vi "JTAG SPI.vi"(4 "Block Write Data":u8[](array[numeric]) format="%02x", 5 "Mask":u8=255 format="%02x", 6 "Blocksize":u16 format="%03x", 7 "Value":u8 format="%02x", 8 "error in (no error)":errorcluster, 9 "Target":u16(ring) items=["Power ASIC", "Stim ASIC", "MICS Radio", "FRAM"], 10 "Function":u16(ring) items=["Power UP", "Power DN", "Write Single", "Read Single", "Write Block", "Read Block", "Write Masked", "Test Value"], 11 "Address":u16 format="%04x") -> (0 "error out":errorcluster, 1 "Block Read Data":u16[](array[numeric]) format="%02x", 2 "Test Result":bool, 3 "Read Value":u8 format="%.0x")   [LabVIEW 2010]
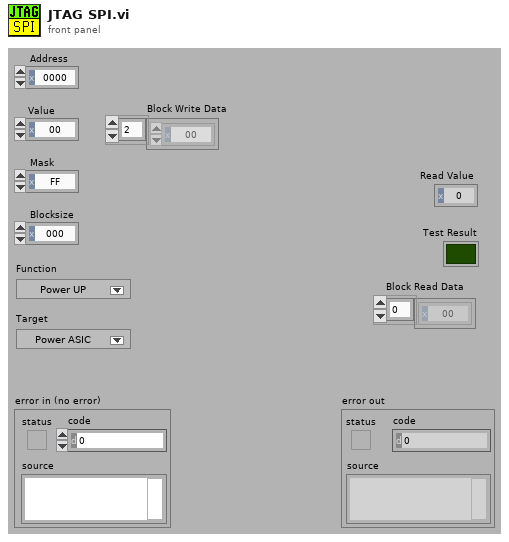
[diagram p1: front panel]
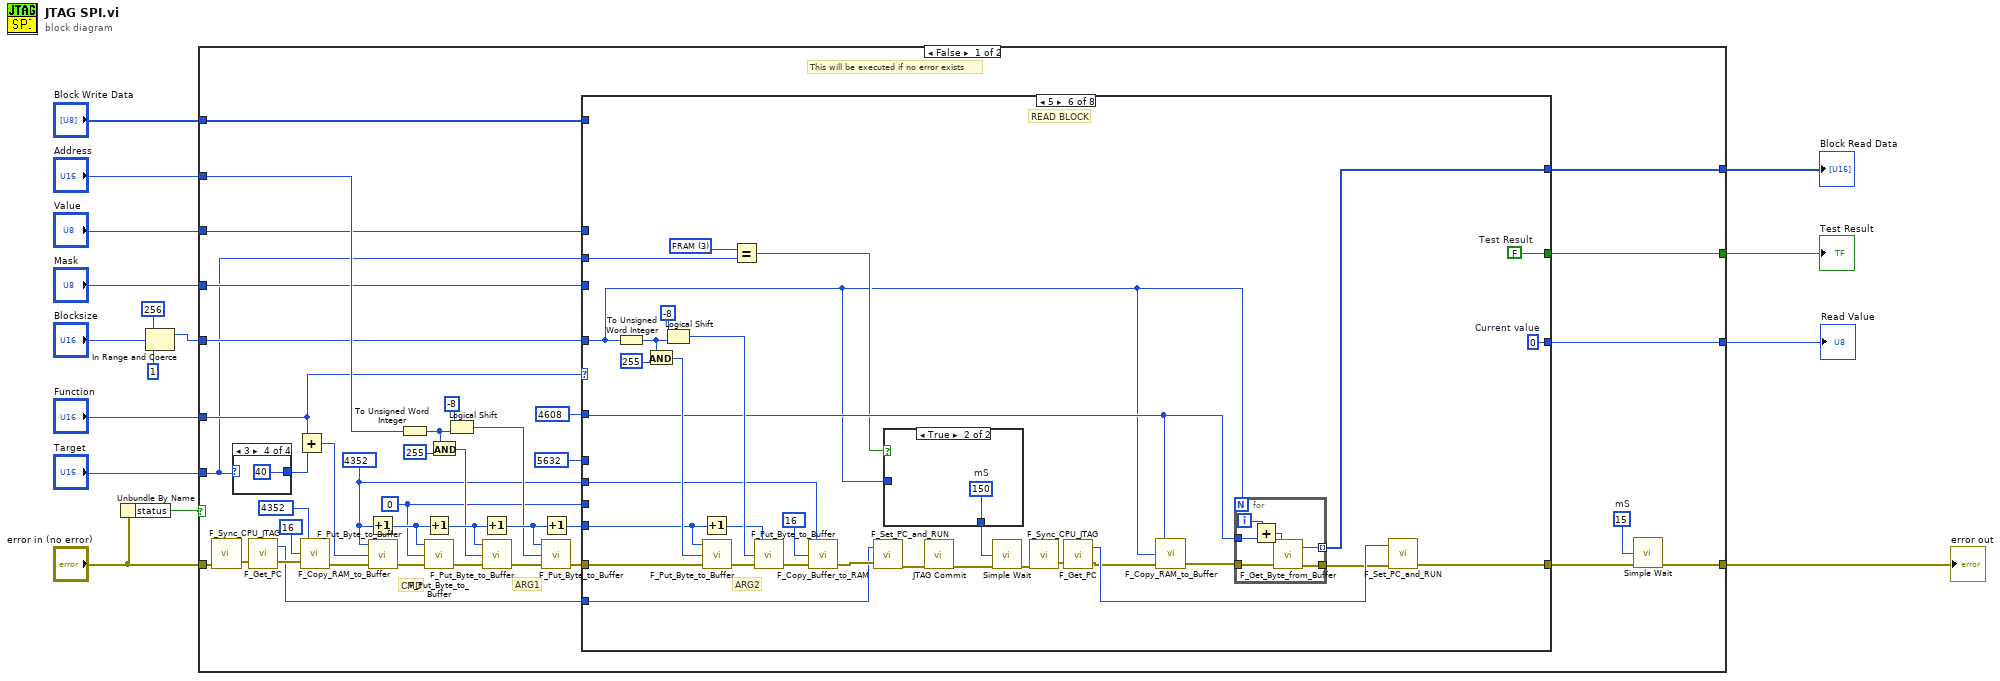
[diagram p0: block diagram]
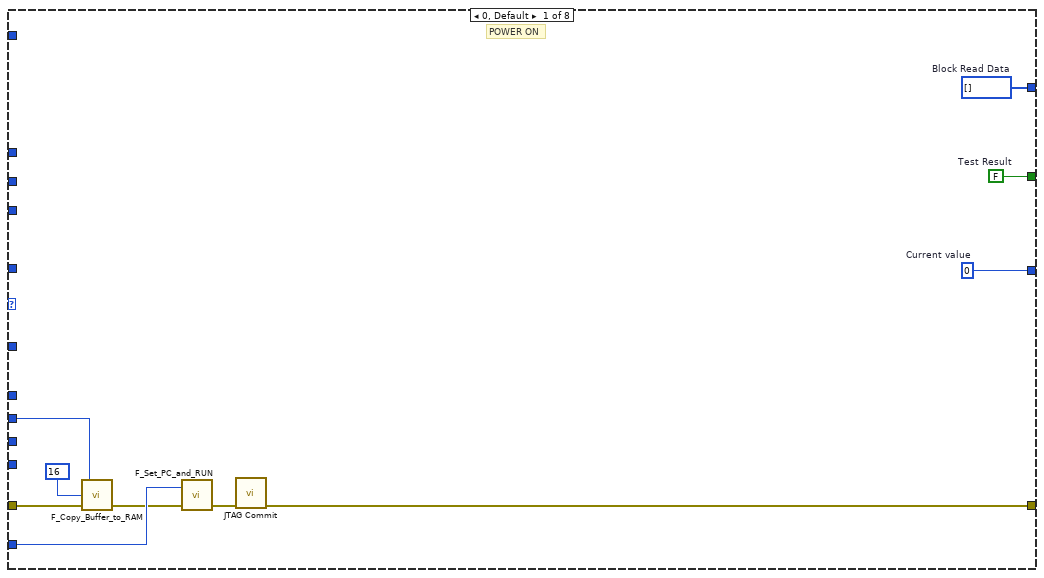
[diagram p2: hidden frame]
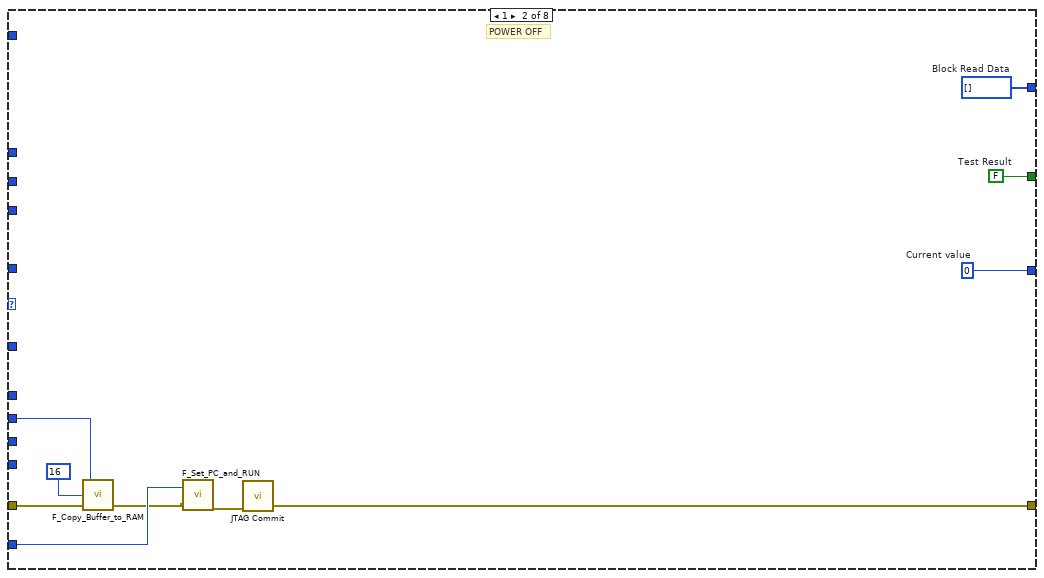
[diagram p3: hidden frame]
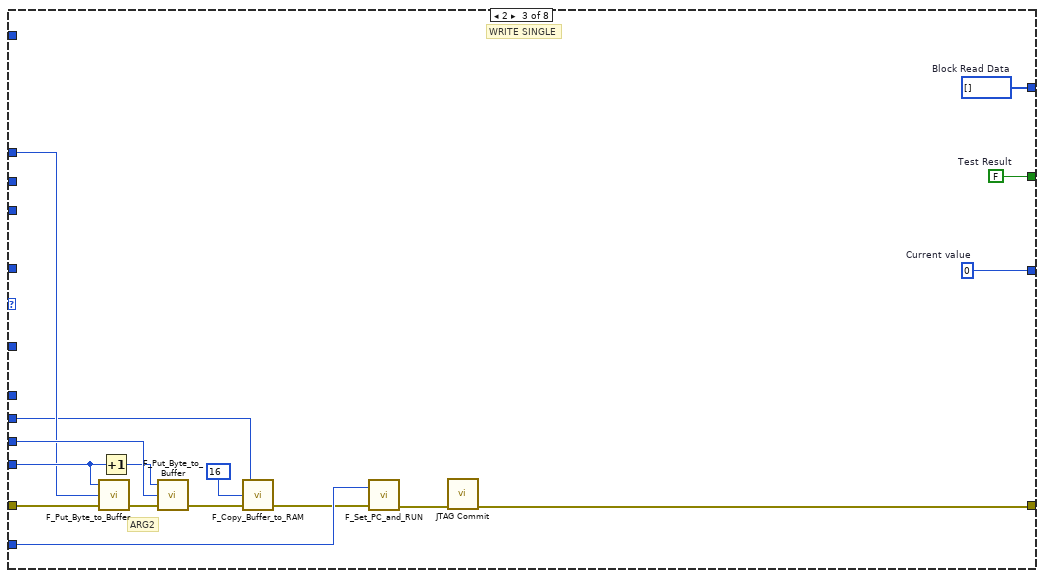
[diagram p4: hidden frame]
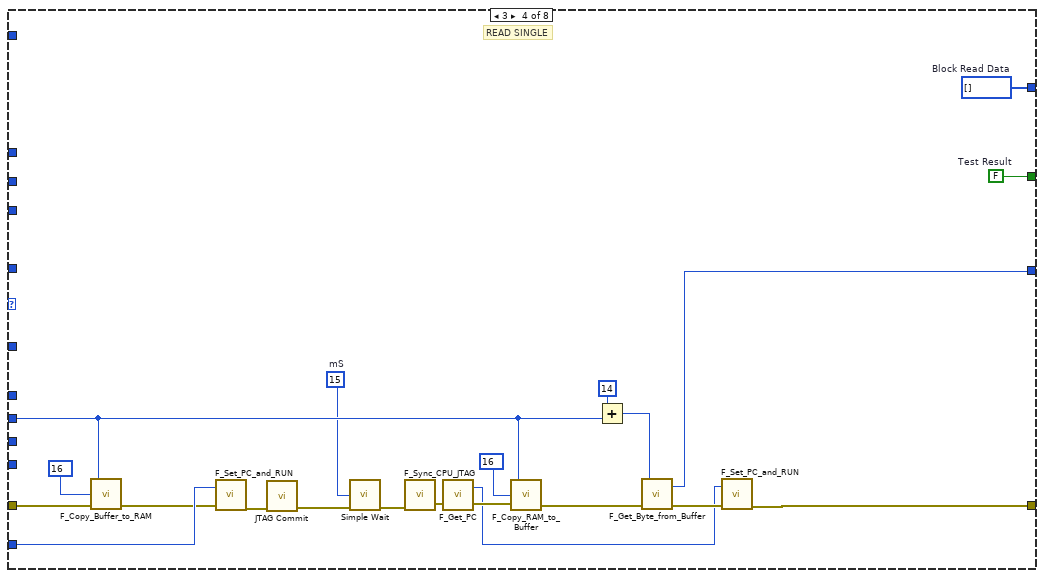
[diagram p5: hidden frame]
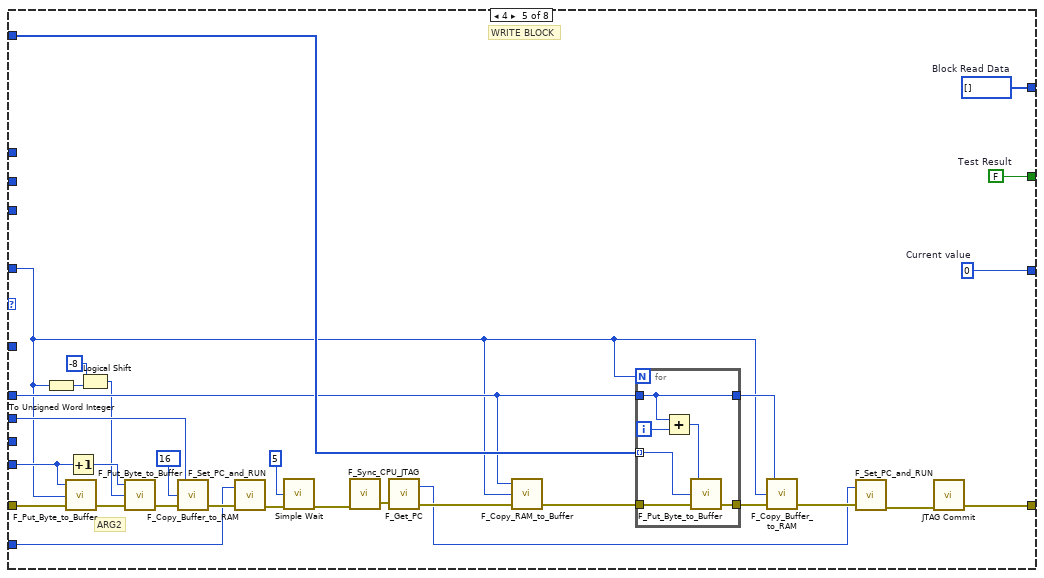
[diagram p6: hidden frame]
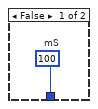
[diagram p7: hidden frame]
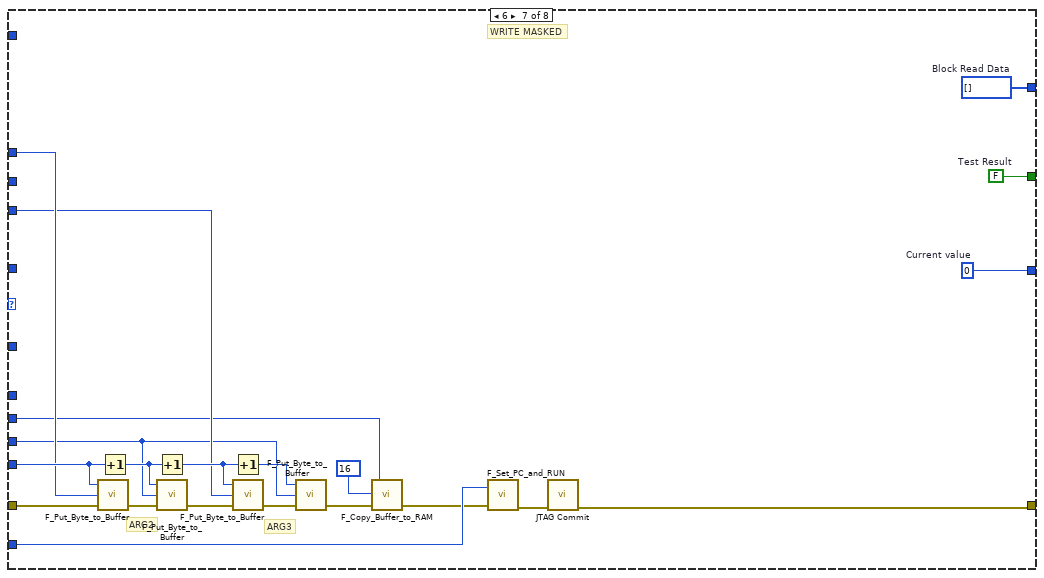
[diagram p8: hidden frame]
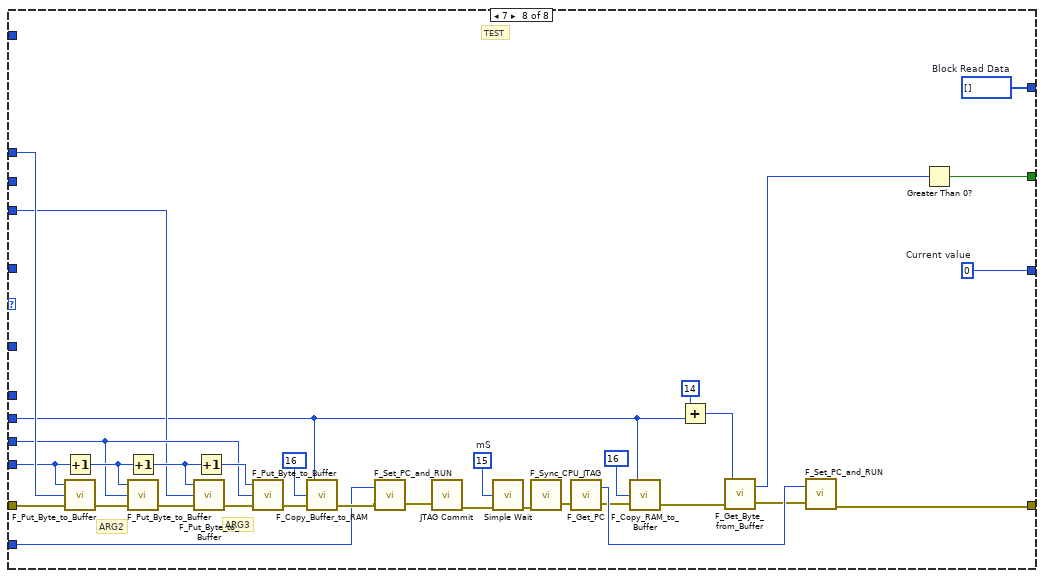
[diagram p9: hidden frame]
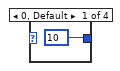
[diagram p10: hidden frame]
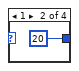
[diagram p11: hidden frame]
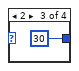
[diagram p12: hidden frame]
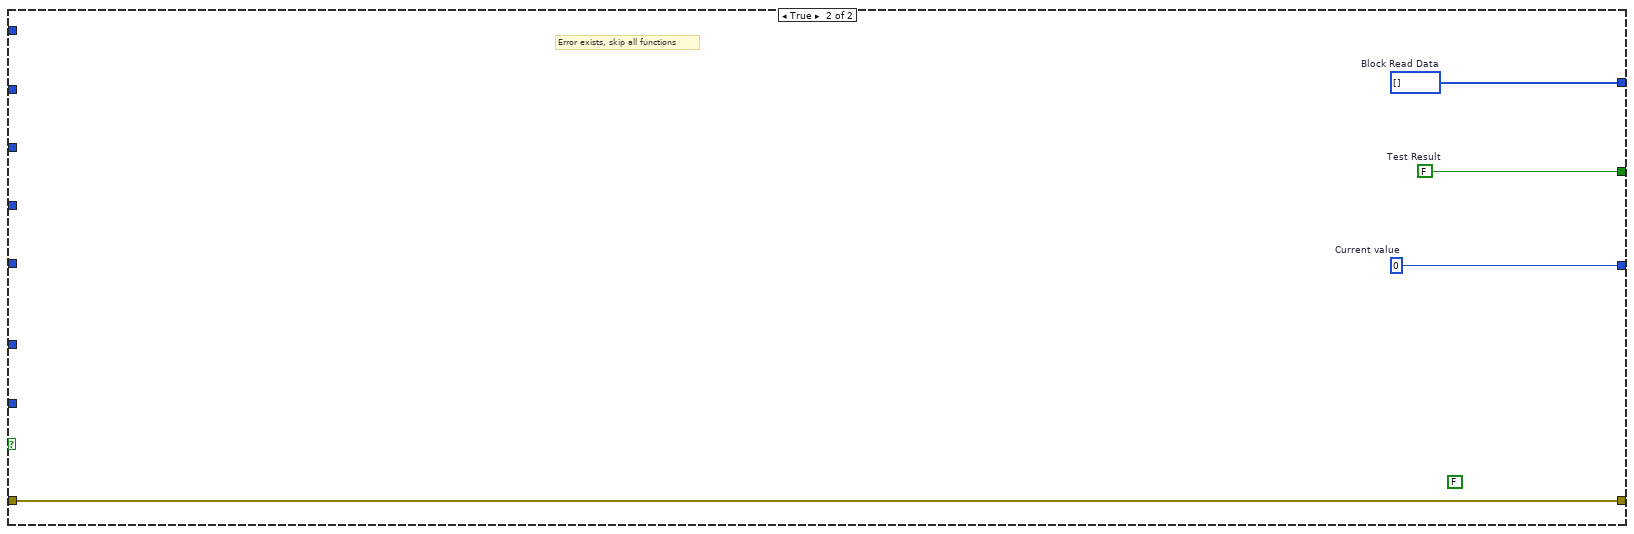
[diagram p13: hidden frame]
diagram:
  n1 = Unbundle By Name("error in (no error)") -> ("status"=w16:bool)
  n2 = In Range and Coerce(upper limit=u16 256, x="Blocksize", lower limit=u16 1) -> (coerced(x)=w4:u16)  [unwired: 1 out]
  n3 = case shown="False" w16 {
    tunnel: [w18 w250] -> w5
    tunnel: "error in (no error)" -> [w55 w250]
    tunnel: "Target" -> [w17 _]
    tunnel: "Address" -> [w44 _]
    tunnel: "Value" -> [w36 _]
    tunnel: "Mask" -> [w33 _]
    tunnel: w4 -> [w29 _]
    tunnel: "Function" -> [w21 _]
    tunnel: "Block Write Data" -> [w37 _]
    tunnel: [w35 w249] -> w7
    tunnel: [w34 w248] -> w8
    tunnel: [w30 w247] -> w6
    frame False {
      w20 = u32 15  # mS
      w38 = u16 0
      w32 = u16 4352
      # "ARG1"
      # "CMD"
      # "This will be executed if no error exists"
      n4 = call "F_Sync_CPU_JTAG.vi"("error in (no error)"=w55) -> ("error out"=w24:errorcluster)  [unwired: 1 in, 1 out]
      n5 = case shown="3" w17 {
        tunnel: [u16 10 u16 20 u16 30 u16 40] -> w54
        frame 0, Default {
        }
        frame 1 {
        }
        frame 2 {
        }
        frame 3 {
        }
      }
      n6 = call "F_Get_PC.vi"("error in (no error)"=w24) -> ("error out"=w23:errorcluster, "Program Counter"=w22:u16)  [unwired: 1 in]
      n7 = Add(x=w21, y=w54) -> (x+y=w53:u16)
      n8 = call "F_Copy_RAM_to_Buffer.vi"("error in (no error)"=w23, "Block size to be copied"=u16 16, "RAM start address"=u16 4352) -> ("error out"=w27:errorcluster)  [unwired: 2 in]
      n9 = Increment(x=w32) -> (x+1=w51:u16)
      n10 = call "F_Put_Byte_to_Buffer.vi"("error in (no error)"=w27, "New value"=w53, "Address of byte to be updated"=w32) -> ("error out"=w52:errorcluster)  [unwired: 2 in]
      n11 = To Unsigned Word Integer(number=w44) -> (unsigned 16bit integer=w41:u16)
      n12 = Increment(x=w51) -> (x+1=w48:u16)
      n13 = call "F_Put_Byte_to_Buffer.vi"("error in (no error)"=w52, "New value"=w38, "Address of byte to be updated"=w51) -> ("error out"=w50:errorcluster)  [unwired: 2 in]
      n14 = And(x=w41, y=u16 255) -> (x .and. y?=w45:u16)
      n15 = Logical Shift(y=i8 -8, x=w41) -> (x << y=w43:u16)
      n16 = Increment(x=w48) -> (x+1=w47:u16)
      n17 = call "F_Put_Byte_to_Buffer.vi"("error in (no error)"=w50, "New value"=w45, "Address of byte to be updated"=w48) -> ("error out"=w49:errorcluster)  [unwired: 2 in]
      n18 = Increment(x=w47) -> (x+1=w40:u16)
      n19 = call "F_Put_Byte_to_Buffer.vi"("error in (no error)"=w49, "New value"=w43, "Address of byte to be updated"=w47) -> ("error out"=w39:errorcluster)  [unwired: 2 in]
      n20 = case shown="5" w21 {
        tunnel: w40 -> [_ _ w87 _ w139 w174 w207 w231]
        tunnel: w39 -> [w60 w70 w89 w105 w141 w178 w208 w234]
        tunnel: w38 -> [_ _ w90 _ _ _ w197 w230]
        tunnel: w29 -> [_ _ _ _ w113 w149 _ _]
        tunnel: w37 -> [_ _ _ _ w134 _ _ _]
        tunnel: w36 -> [_ _ w86 _ _ _ w206 w232]
        tunnel: [w64 w74 w84 w111 w137 w170 w204 w240] -> w35
        tunnel: [w65 w75 w85 w112 w138 w180 w205 w223] -> w34
        tunnel: [w56 w66 w76 w92 w129 w153 w189 w210] -> w19
        tunnel: w33 -> [_ _ _ _ _ _ w198 w229]
        tunnel: w32 -> [w59 w68 w82 w108 w135 w164 w196 w224]
        tunnel: u16 5632 -> [_ _ _ _ w127 _ _ _]
        tunnel: w22 -> [w62 w72 w79 w110 w120 w162 w192 w221]
        tunnel: [w63 w73 w81 w106 w133 w171 w194 w238] -> w30
        tunnel: u16 4608 -> [_ _ _ _ _ w167 _ _]
        tunnel: w17 -> [_ _ _ _ _ w152 _ _]
        frame 0, Default {
          w63 = u8 0  # Current value
          w64 = u16[] []  # Block Read Data
          w65 = FALSE  # Test Result
          # "POWER ON"
          n21 = call "F_Copy_Buffer_to_RAM.vi"("error in (no error)"=w60, "Block size to be copied"=u16 16, "Buffer start address"=w59) -> ("error out"=w58:errorcluster)  [unwired: 2 in]
          n22 = call "F_Set_PC_and_RUN.vi"("error in (no error)"=w58, "PC start address"=w62) -> ("error out"=w57:errorcluster)  [unwired: 1 in]
          n23 = call "JTAG Commit.vi"("error in (no error)"=w57) -> ("error out"=w56:errorcluster)  [unwired: 10 in]
        }
        frame 1 {
          w73 = u8 0  # Current value
          w74 = u16[] []  # Block Read Data
          w75 = FALSE  # Test Result
          # "POWER OFF"
          n24 = call "F_Copy_Buffer_to_RAM.vi"("error in (no error)"=w70, "Block size to be copied"=u16 16, "Buffer start address"=w68) -> ("error out"=w69:errorcluster)  [unwired: 2 in]
          n25 = call "F_Set_PC_and_RUN.vi"("error in (no error)"=w69, "PC start address"=w72) -> ("error out"=w67:errorcluster)  [unwired: 1 in]
          n26 = call "JTAG Commit.vi"("error in (no error)"=w67) -> ("error out"=w66:errorcluster)  [unwired: 10 in]
        }
        frame 2 {
          w81 = u8 0  # Current value
          w84 = u16[] []  # Block Read Data
          w85 = FALSE  # Test Result
          # "WRITE SINGLE"
          # "ARG2"
          n27 = call "F_Put_Byte_to_Buffer.vi"("error in (no error)"=w89, "New value"=w86, "Address of byte to be updated"=w87) -> ("error out"=w91:errorcluster)  [unwired: 2 in]
          n28 = Increment(x=w87) -> (x+1=w88:u16)
          n29 = call "F_Put_Byte_to_Buffer.vi"("error in (no error)"=w91, "New value"=w90, "Address of byte to be updated"=w88) -> ("error out"=w83:errorcluster)  [unwired: 2 in]
          n30 = call "F_Copy_Buffer_to_RAM.vi"("error in (no error)"=w83, "Block size to be copied"=u16 16, "Buffer start address"=w82) -> ("error out"=w78:errorcluster)  [unwired: 2 in]
          n31 = call "F_Set_PC_and_RUN.vi"("error in (no error)"=w78, "PC start address"=w79) -> ("error out"=w77:errorcluster)  [unwired: 1 in]
          n32 = call "JTAG Commit.vi"("error in (no error)"=w77) -> ("error out"=w76:errorcluster)  [unwired: 10 in]
        }
        frame 3 {
          w99 = u32 15  # mS
          w111 = u16[] []  # Block Read Data
          w112 = FALSE  # Test Result
          # "READ SINGLE"
          n33 = call "F_Copy_Buffer_to_RAM.vi"("error in (no error)"=w105, "Block size to be copied"=u16 16, "Buffer start address"=w108) -> ("error out"=w104:errorcluster)  [unwired: 2 in]
          n34 = call "F_Set_PC_and_RUN.vi"("error in (no error)"=w104, "PC start address"=w110) -> ("error out"=w94:errorcluster)  [unwired: 1 in]
          n35 = call "JTAG Commit.vi"("error in (no error)"=w94) -> ("error out"=w93:errorcluster)  [unwired: 10 in]
          n36 = call "Simple Wait.vi"("mS"=w99, "error in"=w93) -> ("error out"=w101:errorcluster)  [unwired: 12 in, 1 out]
          n37 = call "F_Sync_CPU_JTAG.vi"("error in (no error)"=w101) -> ("error out"=w97:errorcluster)  [unwired: 1 in, 1 out]
          n38 = call "F_Get_PC.vi"("error in (no error)"=w97) -> ("error out"=w98:errorcluster, "Program Counter"=w96:u16)  [unwired: 1 in]
          n39 = call "F_Copy_RAM_to_Buffer.vi"("error in (no error)"=w98, "Block size to be copied"=16, "RAM start address"=w108) -> ("error out"=w95:errorcluster)  [unwired: 2 in]
          n40 = Add(x=14 ("Block size to be copied"), y=w108) -> (x+y=w107:i32)
          n41 = call "F_Get_Byte_from_Buffer.vi"("error in (no error)"=w95, "Address of byte to be read"=w107) -> ("error out"=w102:errorcluster, "Current value"=w106:u8)
          n42 = call "F_Set_PC_and_RUN.vi"("error in (no error)"=w102, "PC start address"=w96) -> ("error out"=w92:errorcluster)  [unwired: 1 in]
        }
        frame 4 {
          w133 = u8 0  # Current value
          w137 = u16[] []  # Block Read Data
          w138 = FALSE  # Test Result
          # "WRITE BLOCK"
          # "ARG2"
          n43 = To Unsigned Word Integer(number=w113) -> (unsigned 16bit integer=w115:u16)
          n44 = call "F_Put_Byte_to_Buffer.vi"("error in (no error)"=w141, "New value"=w113, "Address of byte to be updated"=w139) -> ("error out"=w142:errorcluster)  [unwired: 2 in]
          n45 = Increment(x=w139) -> (x+1=w140:u16)
          n46 = Logical Shift(y=i8 -8, x=w115) -> (x << y=w114:u16)
          n47 = call "F_Put_Byte_to_Buffer.vi"("error in (no error)"=w142, "New value"=w114, "Address of byte to be updated"=w140) -> ("error out"=w136:errorcluster)  [unwired: 2 in]
          n48 = call "F_Copy_Buffer_to_RAM.vi"("error in (no error)"=w136, "Block size to be copied"=u16 16, "Buffer start address"=w135) -> ("error out"=w126:errorcluster)  [unwired: 2 in]
          n49 = call "F_Set_PC_and_RUN.vi"("error in (no error)"=w126, "PC start address"=w120) -> ("error out"=w124:errorcluster)  [unwired: 1 in]
          n50 = call "Simple Wait.vi"("mS"=u32 5, "error in"=w124) -> ("error out"=w122:errorcluster)  [unwired: 12 in, 1 out]
          n51 = call "F_Sync_CPU_JTAG.vi"("error in (no error)"=w122) -> ("error out"=w123:errorcluster)  [unwired: 1 in, 1 out]
          n52 = call "F_Get_PC.vi"("error in (no error)"=w123) -> ("error out"=w121:errorcluster, "Program Counter"=w119:u16)  [unwired: 1 in]
          n53 = call "F_Copy_RAM_to_Buffer.vi"("error in (no error)"=w121, "Block size to be copied"=w113, "RAM start address"=w127) -> ("error out"=w128:errorcluster)  [unwired: 2 in]
          n54 = for {
            N: w113 -> [_]
            tunnel: w127 -> [w144]
            tunnel: w134 -> [w146] mode=indexing
            tunnel: w128 -> [w145]
            tunnel: [w144] -> w118
            tunnel: [w143] -> w117
            i -> [w148]
            n55 = Add(x=w144, y=w148) -> (x+y=w147:i32)
            n56 = call "F_Put_Byte_to_Buffer.vi"("error in (no error)"=w145, "New value"=w146, "Address of byte to be updated"=w147) -> ("error out"=w143:errorcluster)  [unwired: 2 in]
          }
          n57 = call "F_Copy_Buffer_to_RAM.vi"("error in (no error)"=w117, "Block size to be copied"=w113, "Buffer start address"=w118) -> ("error out"=w131:errorcluster)  [unwired: 2 in]
          n58 = call "F_Set_PC_and_RUN.vi"("error in (no error)"=w131, "PC start address"=w119) -> ("error out"=w130:errorcluster)  [unwired: 1 in]
          n59 = call "JTAG Commit.vi"("error in (no error)"=w130) -> ("error out"=w129:errorcluster)  [unwired: 10 in]
        }
        frame 5 {
          w151 = u16 3 items=["Power ASIC", "Stim ASIC", "MICS Radio", "FRAM"] ("Target")
          w171 = u8 0  # Current value
          w180 = FALSE  # Test Result
          # "READ BLOCK"
          # "ARG2"
          n60 = To Unsigned Word Integer(number=w149) -> (unsigned 16bit integer=w176:u16)
          n61 = And(x=w176, y=u16 255) -> (x .and. y?=w175:u16)
          n62 = Logical Shift(y=i8 -8, x=w176) -> (x << y=w173:u16)
          n63 = Increment(x=w174) -> (x+1=w172:u16)
          n64 = call "F_Put_Byte_to_Buffer.vi"("error in (no error)"=w178, "New value"=w175, "Address of byte to be updated"=w174) -> ("error out"=w179:errorcluster)  [unwired: 2 in]
          n65 = Equal?(x=w151, y=w152) -> (x = y?=w150:bool)
          n66 = call "F_Put_Byte_to_Buffer.vi"("error in (no error)"=w179, "New value"=w173, "Address of byte to be updated"=w172) -> ("error out"=w166:errorcluster)  [unwired: 2 in]
          n67 = call "F_Copy_Buffer_to_RAM.vi"("error in (no error)"=w166, "Block size to be copied"=u16 16, "Buffer start address"=w164) -> ("error out"=w165:errorcluster)  [unwired: 2 in]
          n68 = call "F_Set_PC_and_RUN.vi"("error in (no error)"=w165, "PC start address"=w162) -> ("error out"=w155:errorcluster)  [unwired: 1 in]
          n69 = case shown="True" w150 {
            tunnel: [w181 w182] -> w159
            tunnel: w149 -> [_ _]
            frame False {
              w181 = u32 100  # mS
            }
            frame True {
              w182 = u32 150  # mS
            }
          }
          n70 = call "JTAG Commit.vi"("error in (no error)"=w155) -> ("error out"=w154:errorcluster)  [unwired: 10 in]
          n71 = call "Simple Wait.vi"("mS"=w159, "error in"=w154) -> ("error out"=w158:errorcluster)  [unwired: 12 in, 1 out]
          n72 = call "F_Sync_CPU_JTAG.vi"("error in (no error)"=w158) -> ("error out"=w157:errorcluster)  [unwired: 1 in, 1 out]
          n73 = call "F_Get_PC.vi"("error in (no error)"=w157) -> ("error out"=w156:errorcluster, "Program Counter"=w161:u16)  [unwired: 1 in]
          n74 = call "F_Copy_RAM_to_Buffer.vi"("error in (no error)"=w156, "Block size to be copied"=w149, "RAM start address"=w167) -> ("error out"=w168:errorcluster)  [unwired: 2 in]
          n75 = for {
            N: w149 -> [_]
            tunnel: w168 -> [w188]
            tunnel: [w187] -> w160
            tunnel: w167 -> [w186]
            tunnel: [w183] -> w170 mode=indexing
            i -> [w185]
            n76 = Add(x=w185, y=w186) -> (x+y=w184:i32)
            n77 = call "F_Get_Byte_from_Buffer.vi"("error in (no error)"=w188, "Address of byte to be read"=w184) -> ("error out"=w187:errorcluster, "Current value"=w183:u8)
          }
          n78 = call "F_Set_PC_and_RUN.vi"("error in (no error)"=w160, "PC start address"=w161) -> ("error out"=w153:errorcluster)  [unwired: 1 in]
        }
        frame 6 {
          w194 = u8 0  # Current value
          w204 = u16[] []  # Block Read Data
          w205 = FALSE  # Test Result
          # "WRITE MASKED"
          # "ARG3"
          # "ARG2"
          n79 = call "F_Put_Byte_to_Buffer.vi"("error in (no error)"=w208, "New value"=w206, "Address of byte to be updated"=w207) -> ("error out"=w209:errorcluster)  [unwired: 2 in]
          n80 = Increment(x=w207) -> (x+1=w203:u16)
          n81 = Increment(x=w203) -> (x+1=w199:u16)
          n82 = call "F_Put_Byte_to_Buffer.vi"("error in (no error)"=w209, "New value"=w197, "Address of byte to be updated"=w203) -> ("error out"=w200:errorcluster)  [unwired: 2 in]
          n83 = Increment(x=w199) -> (x+1=w201:u16)
          n84 = call "F_Put_Byte_to_Buffer.vi"("error in (no error)"=w200, "New value"=w198, "Address of byte to be updated"=w199) -> ("error out"=w202:errorcluster)  [unwired: 2 in]
          n85 = call "F_Put_Byte_to_Buffer.vi"("error in (no error)"=w202, "New value"=w197, "Address of byte to be updated"=w201) -> ("error out"=w195:errorcluster)  [unwired: 2 in]
          n86 = call "F_Copy_Buffer_to_RAM.vi"("error in (no error)"=w195, "Block size to be copied"=u16 16, "Buffer start address"=w196) -> ("error out"=w191:errorcluster)  [unwired: 2 in]
          n87 = call "F_Set_PC_and_RUN.vi"("error in (no error)"=w191, "PC start address"=w192) -> ("error out"=w190:errorcluster)  [unwired: 1 in]
          n88 = call "JTAG Commit.vi"("error in (no error)"=w190) -> ("error out"=w189:errorcluster)  [unwired: 10 in]
        }
        frame 7 {
          w218 = u32 15  # mS
          w238 = u8 0  # Current value
          w240 = u16[] []  # Block Read Data
          # "TEST"
          # "ARG2"
          # "ARG3"
          n89 = Increment(x=w231) -> (x+1=w236:u16)
          n90 = call "F_Put_Byte_to_Buffer.vi"("error in (no error)"=w234, "New value"=w232, "Address of byte to be updated"=w231) -> ("error out"=w237:errorcluster)  [unwired: 2 in]
          n91 = Increment(x=w236) -> (x+1=w235:u16)
          n92 = call "F_Put_Byte_to_Buffer.vi"("error in (no error)"=w237, "New value"=w230, "Address of byte to be updated"=w236) -> ("error out"=w233:errorcluster)  [unwired: 2 in]
          n93 = call "F_Put_Byte_to_Buffer.vi"("error in (no error)"=w233, "New value"=w229, "Address of byte to be updated"=w235) -> ("error out"=w242:errorcluster)  [unwired: 2 in]
          n94 = Increment(x=w235) -> (x+1=w241:u16)
          n95 = call "F_Put_Byte_to_Buffer.vi"("error in (no error)"=w242, "New value"=w230, "Address of byte to be updated"=w241) -> ("error out"=w239:errorcluster)  [unwired: 2 in]
          n96 = call "F_Copy_Buffer_to_RAM.vi"("error in (no error)"=w239, "Block size to be copied"=u16 16, "Buffer start address"=w224) -> ("error out"=w228:errorcluster)  [unwired: 2 in]
          n97 = call "F_Set_PC_and_RUN.vi"("error in (no error)"=w228, "PC start address"=w221) -> ("error out"=w212:errorcluster)  [unwired: 1 in]
          n98 = call "JTAG Commit.vi"("error in (no error)"=w212) -> ("error out"=w211:errorcluster)  [unwired: 10 in]
          n99 = call "Simple Wait.vi"("mS"=w218, "error in"=w211) -> ("error out"=w217:errorcluster)  [unwired: 12 in, 1 out]
          n100 = call "F_Sync_CPU_JTAG.vi"("error in (no error)"=w217) -> ("error out"=w215:errorcluster)  [unwired: 1 in, 1 out]
          n101 = call "F_Get_PC.vi"("error in (no error)"=w215) -> ("error out"=w214:errorcluster, "Program Counter"=w220:u16)  [unwired: 1 in]
          n102 = call "F_Copy_RAM_to_Buffer.vi"("error in (no error)"=w214, "Block size to be copied"=16, "RAM start address"=w224) -> ("error out"=w213:errorcluster)  [unwired: 2 in]
          n103 = Add(x=14 ("Block size to be copied"), y=w224) -> (x+y=w226:i32)
          n104 = call "F_Get_Byte_from_Buffer.vi"("error in (no error)"=w213, "Address of byte to be read"=w226) -> ("error out"=w219:errorcluster, "Current value"=w225:u8)
          n105 = call "F_Set_PC_and_RUN.vi"("error in (no error)"=w219, "PC start address"=w220) -> ("error out"=w210:errorcluster)  [unwired: 1 in]
          n106 = Greater Than 0?(x=w225) -> (x > 0?=w223:bool)
        }
      }
      n107 = call "Simple Wait.vi"("mS"=w20, "error in"=w19) -> ("error out"=w18:errorcluster)  [unwired: 12 in, 1 out]
    }
    frame True {
      (unwired) FALSE
      w247 = u8 0  # Current value
      w249 = u16[] []  # Block Read Data
      w248 = FALSE  # Test Result
      # "Error exists, skip all functions"
    }
  }
  "error out" <- w5
  "Test Result" <- w8
  "Block Read Data" <- w7
  "Read Value" <- w6
